vi "fitting_1d_pixel.vi"(6 "D sign":dbl, 7 "side velocity threshold":dbl, 8 "fitting axis":dbl, 9 "ratio_pixel2mil":dbl, 11 "array in":dbl[][](array[numeric])) -> (0 "D":ext[](array[numeric]), 2 "slope":dbl, 3 "fitting array":dbl[][](array[numeric]))   [LabVIEW 2017]
uses:
  <vilib>/Analysis/NI_AALPro.lvlib
panel:
  out "Array out 2":ext[](array[numeric])
  out "Array out":ext[](array[numeric])
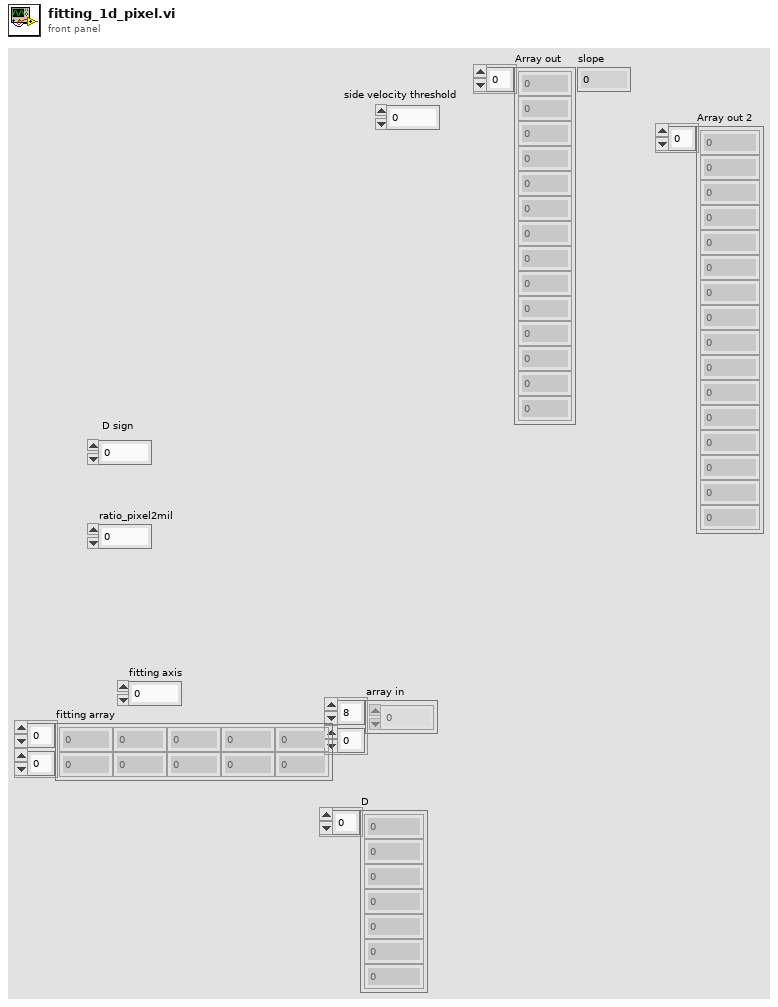
[diagram p1: front panel]
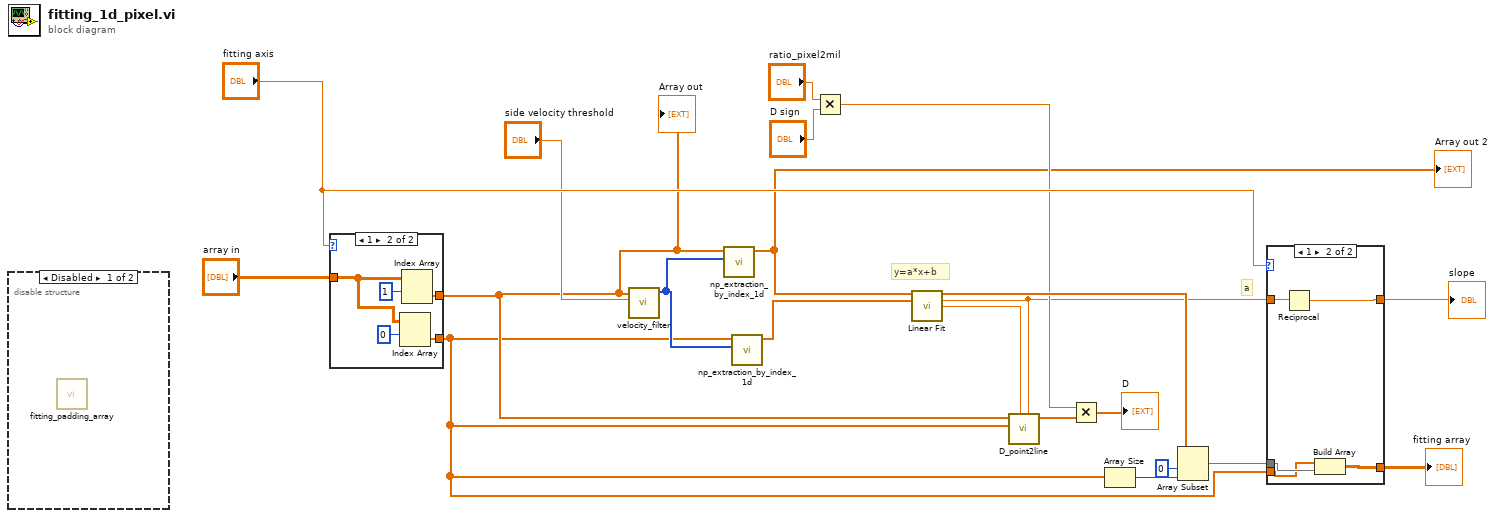
[diagram p0: block diagram]
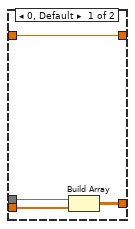
[diagram p3: hidden frame]
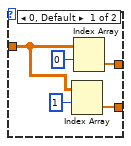
[diagram p4: hidden frame]
diagram:
  # "a"
  # "y=a*x+b"
  n1 = disable-structure shown="Disabled" {
    frame Disabled {
      n2 = call "fitting_padding_array.vi"() -> ()  [unwired: 11 in, 1 out]
    }
    frame Enabled {
    }
  }
  n3 = case shown="1" "fitting axis" {
    tunnel: "array in" -> [w24 w29]
    tunnel: [w23 w28] -> w3
    tunnel: [w22 w27] -> w2
    frame 0, Default {
      n4 = Index Array(array=w24, index (row)=1) -> (element=w22:dbl[])  [unwired: 1 in]
      n5 = Index Array(array=w24, index (row)=0) -> (element=w23:dbl[])  [unwired: 1 in]
    }
    frame 1 {
      n6 = Index Array(array=w29, index (row)=0) -> (element=w27:dbl[])  [unwired: 1 in]
      n7 = Index Array(array=w29, index (row)=1) -> (element=w28:dbl[])  [unwired: 1 in]
    }
  }
  "Array out" <- w3
  n8 = call "velocity_filter.vi"("threshold"="side velocity threshold", "Array in"=w3) -> ("index"=w9:i32[])  [unwired: 9 in]
  n9 = call "np_extraction_by_index_1d.vi"("index array"=w9, "Array in"=w3) -> ("Array out"=w7:ext[])  [unwired: 9 in]
  "Array out 2" <- w7
  n10 = call "np_extraction_by_index_1d.vi"("index array"=w9, "Array in"=w2) -> ("Array out"=w8:ext[])  [unwired: 9 in]
  n11 = Multiply(x="ratio_pixel2mil", y="D sign") -> (x*y=w11:dbl)
  n12 = call <vilib>:"Linear Fit.vi"("Y"=w7, "X"=w8) -> ("Best Linear Fit"=w20:dbl[], "slope"=w6:dbl, "intercept"=w5:dbl)  [unwired: 9 in, 2 out]
  n13 = call "D_point2line.vi"("slope"=w6, "intercept"=w5, "X Array"=w2, "Y Array"=w3) -> ("D"=w16:ext[])  [unwired: 5 in, 2 out]
  n14 = Multiply(x=w11, y=w16) -> (x*y=→"D":ext[])
  n15 = Array Size(array=w2) -> (size(s)=w21:i32)
  n16 = Array Subset(array=w20, index=0, length=w21) -> (w19:dbl[])
  n17 = case shown="1" "fitting axis" {
    tunnel: w19 -> [w35 w39]
    tunnel: w2 -> [w34 w38]
    tunnel: [w33 w40] -> w15
    tunnel: w6 -> [w32 w37]
    tunnel: [w32 w36] -> w4
    frame 0, Default {
      n18 = Build Array(w35, w34) -> (w33:dbl[][])
    }
    frame 1 {
      n19 = Reciprocal(x=w37) -> (1/x=w36:dbl)
      n20 = Build Array(w38, w39) -> (w40:dbl[][])
    }
  }
  "fitting array" <- w15
  "slope" <- w4
